vi "Config Input.vi"(0 "VISA resource name":refnum<visa-resource-name>, 5 "Input Group (0:Inputs 1-4)":u16(ring) items=["Inputs 1-4", "Inputs 5-8"], 7 "Sensor Type (0:2.5V Diode)":u16(ring) items=["2.5V Diode", "7.5V Diode", "250 Ohm Platinum", "500 Ohm Platinum", "5K Ohm Platinum", "Cernox"], 9 "Input (1)":dbl=1.0 min=1.0 max=8.0 step=1.0, 11 "error in (no error)":errorcluster, 12 "Input (T: Input ON)":bool=TRUE, 13 "Input Curve (0:None)":u16(ring) items=["None", "DT-470", "DT-500", "CTI Diode", "Empty Standard Diode", "Empty Standard Diode", "PT-100", "PT-1000", "Empty Standard Platinum", "Empty Standard Platinum", "Unused", "Unused", "Unused", "Unused", "Unused", "Unused", "Unused", "Unused", "Unused", "Unused", "Unused", "User Curve 1", "User Curve 2", "User Curve 3", "User Curve 4", "User Curve 5", "User Curve 6", "User Curve 7", "User Curve 8"]) -> (4 "VISA resource name out":refnum<visa-resource-name>, 15 "error out":errorcluster)   [LabVIEW 2017, in "Lake Shore Cryotronics 218.lvlib"]
doc: "This VI configures the following parameters of the 218 inputs:\n\nSensor type for each input group.\nTurns individual inputs on and off.\nSelects Curve for individual inputs."
uses:
  Lake Shore Cryotronics 218.lvlib
panel:
  # "Input ON\nInput OFF"
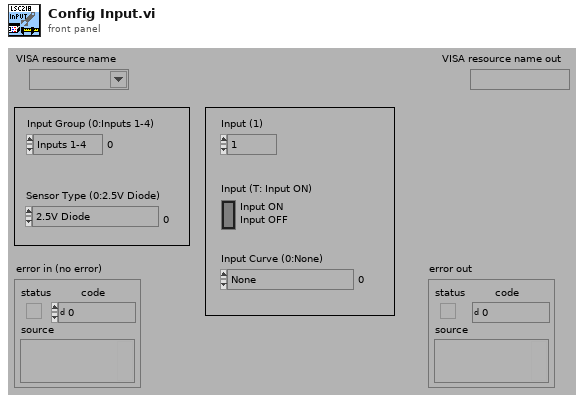
[diagram p1: front panel]
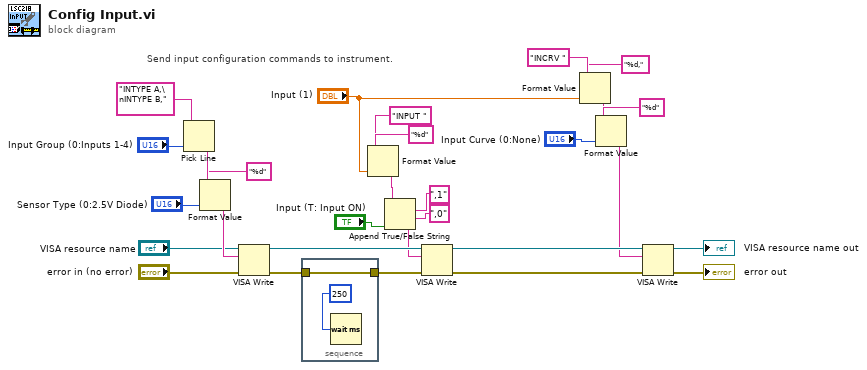
[diagram p0: block diagram]
diagram:
  # "Send input configuration commands to instrument."
  n1 = Pick Line(multi-line string="INTYPE A,\nINTYPE B,", line index="Input Group (0:Inputs 1-4)") -> (output string=w24:string)  [unwired: 1 in]
  n2 = Format Value(string ("")=w24, format string="%d", value (0)="Sensor Type (0:2.5V Diode)") -> (output string=w21:string)
  n3 = VISA Write(VISA resource name="VISA resource name", write buffer=w21, error in (no error)="error in (no error)") -> (VISA resource name out=w20:refnum<visa-resource-name>, error out=w7:errorcluster)  [unwired: 1 out]
  n4 = stacked-sequence {
    tunnel: w7 -> [w31]
    tunnel: [w31] -> w6
    frame #0 {
      n5 = Wait (ms)(milliseconds to wait=u32 250) -> ()  [unwired: 1 out]
    }
  }
  n6 = Format Value(string ("")="INPUT ", format string="%d", value (0)="Input (1)") -> (output string=w16:string)
  n7 = Append True/False String(1:"Input (T: Input ON)", 2:",0", 3:",1", 4:w16) -> (0:w15:string)
  n8 = VISA Write(VISA resource name=w20, write buffer=w15, error in (no error)=w6) -> (VISA resource name out=w19:refnum<visa-resource-name>, error out=w5:errorcluster)  [unwired: 1 out]
  n9 = Format Value(string ("")="INCRV ", format string="%d,", value (0)="Input (1)") -> (output string=w10:string)
  n10 = Format Value(string ("")=w10, format string="%d", value (0)="Input Curve (0:None)") -> (output string=w8:string)
  n11 = VISA Write(VISA resource name=w19, write buffer=w8, error in (no error)=w5) -> (VISA resource name out=→"VISA resource name out":refnum<visa-resource-name>, error out=→"error out":errorcluster)  [unwired: 1 out]
